vi "nivsfpga_CreateConditionalSymbol.vi"(8 "error in (no error)":errorcluster, 9 "New Value":string="Test,1;", 10 "New Symbol":string="Test,1;", 11 "reference":refnum<vi>) -> (0 "error out":errorcluster, 3 "reference out":refnum<vi>)   [LabVIEW 2010]
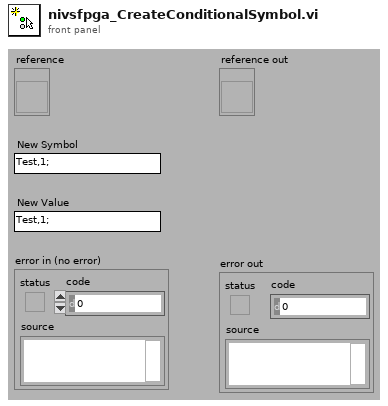
[diagram p1: front panel]
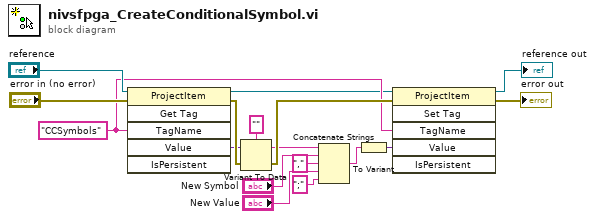
[diagram p0: block diagram]
diagram:
  w3 = "CCSymbols" ("Tag Name")
  n1 = invoke class="ProjectItem" method="Get Tag"(reference="reference", error in="error in (no error)", "TagName"=w3) -> (reference out=w1:refnum<vi>, error out=w12:errorcluster, "Value"=w2:variant)  [unwired: 3 in, 3 out]
  n2 = Variant To Data(error in=w12, Variant=w2, type="" ("Tag Name")) -> (error out=w13:errorcluster, data=w5:string)
  n3 = Concatenate Strings(w5, "New Symbol", "," ("string"), "New Value", ";" ("string")) -> (w7:string)
  n4 = To Variant(anything=w7) -> (Variant=w6:variant)
  n5 = invoke class="ProjectItem" method="Set Tag"(reference=w1, error in=w13, "TagName"=w3, "Value"=w6) -> (reference out=→"reference out":refnum<vi>, error out=→"error out":errorcluster)  [unwired: 2 in, 4 out]
